vi "Volts_to_mW.vi"(11 "Volts":dbl[](array[numeric])) -> (3 "Power mW":dbl[](array[numeric]))   [LabVIEW 2018]
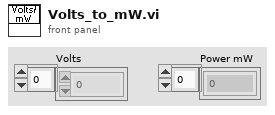
[diagram p1: front panel]
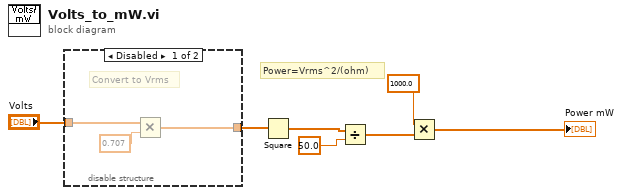
[diagram p0: block diagram]
diagram:
  # "Power=Vrms^2/(ohm)"
  n1 = disable-structure shown="Disabled" {
    disable-tunnel: [w10 w11] -> w5
    disable-tunnel: "Volts" -> [w8 w11]
    frame Disabled {
      # "Convert to Vrms"
      n2 = Multiply(x=w8, y=0.707) -> (x*y=w10:dbl[])
    }
    frame Enabled {
      # "No longer convewrrt to Vrms.\nInherent to FFT\n12-15-2020"
    }
  }
  n3 = Square(x=w5) -> (x^2=w4:dbl[])
  n4 = Divide(x=w4, y=50.0) -> (x/y=w1:dbl[])
  n5 = Multiply(x=1000.0, y=w1) -> (x*y=→"Power mW":dbl[])
